vi "TA Main.vi"() -> ()   [LabVIEW 2019]
doc: "This example demonstrates how to acquire a continuous amount of data (Waveform) using the DAQ device's internal clock. It also shows how to synchronize two devices for different device families (E Series, S Series, M Series, X Series, DSA, and SC Express), to simultaneously acquire the data.\n\nFor instructions on how to connect your signals to the DAQ device, refer to your device documentation."
uses:
  <vilib>/Utility/error.llb/DialogType.ctl
  <vilib>/DAQmx/configure/trigger.llb/DAQmx Start Trigger (Digital Edge).vi
  <vilib>/DAQmx/read.llb/DAQmx Read (Analog 1D Wfm NChan NSamp).vi
  <vilib>/DAQmx/configure/timing.llb/DAQmx Timing (Sample Clock).vi
  <vilib>/Instr/_visa.llb/VISA Configure Serial Port (Instr).vi
  Program Files/National Instruments/LabVIEW 2019/examples/Instrument IO/Serial/support/Serial - Settings.ctl
panel:
  in  "Pass Logger":T1(tab)
  out "CO2 chart":waveform(dbl)[](graph)=[{"t0"=timestamp(3654846988.5963 s since 1904-01-01), "dt"=0.0, "Y"=[566.0], "attributes"=variant("NI_ChannelName"=variant(string "SCD30 CO2"), "NI_UnitDescription"=variant(string "ppm"))}, {"t0"=timestamp(3654846988.5963 s since 1904-01-01), "dt"=0.0, "Y"=[28.99], "attributes"=variant("NI_ChannelName"=variant(string "SCD30 Temp"), "NI_UnitDescription"=variant(string "C"))}, {"t0"=timestamp(3654846988.5963 s since 1904-01-01), "dt"=0.0, "Y"=[22.24], "attributes"=variant("NI_ChannelName"=variant(string "SCD30 Humidity"), "NI_UnitDescription"=variant(string "%"))}, {"t0"=timestamp(3654846988.5963 s since 1904-01-01), "dt"=0.0, "Y"=[28.2], "attributes"=variant("NI_ChannelName"=variant(string "BME680 Temp"), "NI_UnitDescription"=variant(string "C"))}, {"t0"=timestamp(3654846988.5963 s since 1904-01-01), "dt"=0.0, "Y"=[1011.41], "attributes"=variant("NI_ChannelName"=variant(string "hPa"), "NI_UnitDescription"=variant(string "BME680 Pressure"))}, {"t0"=timestamp(3654846988.5963 s since 1904-01-01), "dt"=0.0, "Y"=[23.86], "attributes"=variant("NI_ChannelName"=variant(string "BME680 Humidity"), "NI_UnitDescription"=variant(string "%"))}, {"t0"=timestamp(3654846988.5963 s since 1904-01-01), "dt"=0.0, "Y"=[407.63], "attributes"=variant("NI_ChannelName"=variant(string "BME680 Gas"), "NI_UnitDescription"=variant(string "KOhms"))}]
  in  "Stop":bool
  in  "Enable logging":bool=TRUE caption="Enable"
  in  "File config":T2={"Filepath"=path "C:/Users/Administrator/Desktop/DAQ PAS/Test data", "Test ID"="CO2_oven_V3_1v2_25C", "PC"="69DTQV2"}
  out "Lockin chart":waveform(dbl)[](graph)=[{"t0"=timestamp(3654846973.919467 s since 1904-01-01), "dt"=9.999, "Y"=[0.5432839233173321], "attributes"=variant("NI_ChannelName"=variant(string "Phase - Mic Diff"), "NI_UnitDescription"=variant(string "Rad"))}, {"t0"=timestamp(3654846973.919467 s since 1904-01-01), "dt"=9.999, "Y"=[0.28139672074027666], "attributes"=variant("NI_ChannelName"=variant(string "Amplitude - Mic Diff"), "NI_UnitDescription"=variant(string "Volts"))}]
  out "Lockin output 1":T3={"X"=0.12044000212072635, "Y"=0.07273399824019537, "R"=0.14069836037013833, "θ"=0.5432839233173321, "Amp"=0.28139672074027666, "dt"=9.999, "Active channel"="Mic Diff", "Ref channel"="Heater Voltage"} {"X" format="%#_3g"; "Y" format="%#_3g"; "R" format="%#_3g"}
  out "Reference sesnsor readings":T4={"SCD30 CO2"=566.0, "SCD30 Temp (C)"=28.99, "SCD30 RH (%)"=22.24, "BME680 Temp (C) "=28.2, "BME680 Presssure (hPa)"=1011.41, "BME680 RH (%) "=23.86, "BME680 Gas (KOhms)"=407.63}
  in  "Sampling config":cluster{"Fs":dbl, "#s":dbl}={"Fs"=1000.0, "#s"=10000.0} {"Fs" format="%.2p"}
  in  "Config 1":cluster{"Ref Index":i32, "Active Index":i32}={"Ref Index"=2, "Active Index"=4}
  out "Lockin output 5":T3={"X"=4.105476127421498, "Y"=0.07771898305094777, "R"=4.106211693660507, "θ"=0.018928304216159014, "Amp"=8.212423387321014, "dt"=9.999, "Active channel"="Heater Current", "Ref channel"="Heater Voltage"} {"X" format="%#_3g"; "Y" format="%#_3g"; "R" format="%#_3g"}
  out "Lockin output 6":T3={"X"=5.873296336618479, "Y"=0.05854532299570415, "R"=5.873588120781088, "θ"=0.009967721820028476, "Amp"=11.747176241562176, "dt"=9.999, "Active channel"="Heater Power", "Ref channel"="Heater Voltage"} {"X" format="%#_3g"; "Y" format="%#_3g"; "R" format="%#_3g"}
  out "Lockin output 4":T3={"X"=0.31867008645671724, "Y"=3.873316981852211e-05, "R"=0.31867008881065395, "θ"=0.00012154629905321044, "Amp"=0.6373401776213079, "dt"=9.999, "Active channel"="Heater Voltage", "Ref channel"="Heater Voltage"} {"X" format="%#_3g"; "Y" format="%#_3g"; "R" format="%#_3g"}
  out "Lockin output 3":T3={"X"=-0.12845683117209084, "Y"=-0.046514562917248106, "R"=0.1366190398083579, "θ"=-2.7941768834347642, "Amp"=0.2732380796167158, "dt"=9.999, "Active channel"="Mic Active", "Ref channel"="Heater Voltage"} {"X" format="%#_3g"; "Y" format="%#_3g"; "R" format="%#_3g"}
  out "Lockin output 2":T3={"X"=-0.008448931381000458, "Y"=0.02761458480398332, "R"=0.02887818788250469, "θ"=1.8677111087244906, "Amp"=0.05775637576500938, "dt"=9.999, "Active channel"="Mic Ref", "Ref channel"="Heater Voltage"} {"X" format="%#_3g"; "Y" format="%#_3g"; "R" format="%#_3g"}
  in  "Config 5":cluster{"Ref Index":i32, "Active Index":i32}={"Ref Index"=2, "Active Index"=5}
  in  "Config 4":cluster{"Ref Index":i32, "Active Index":i32}={"Ref Index"=2, "Active Index"=2}
  in  "Config 3":cluster{"Ref Index":i32, "Active Index":i32}={"Ref Index"=2, "Active Index"=1}
  in  "Config 2":cluster{"Ref Index":i32, "Active Index":i32}={"Ref Index"=2, "Active Index"=0}
  in  "Config 6":cluster{"Ref Index":i32, "Active Index":i32}={"Ref Index"=2, "Active Index"=7}
  out "Lockin output 1":T3={"X"=0.12044000212072635, "Y"=0.07273399824019537, "R"=0.14069836037013833, "θ"=0.5432839233173321, "Amp"=0.28139672074027666, "dt"=9.999, "Active channel"="Mic Diff", "Ref channel"="Heater Voltage"} {"X" format="%#_3g"; "Y" format="%#_3g"; "R" format="%#_3g"}
  in  "Config 7":cluster{"Ref Index":i32, "Active Index":i32}={"Ref Index"=2, "Active Index"=6}
  out "Lockin output 7":T3={"X"=7.678486794988711, "Y"=-0.3885980124293869, "R"=7.6883137212317285, "θ"=-0.05056553039103557, "Amp"=15.376627442463457, "dt"=9.999, "Active channel"="Heater Resistance", "Ref channel"="Heater Voltage"} {"X" format="%#_3g"; "Y" format="%#_3g"; "R" format="%#_3g"}
  in  "VISA resource name 2":refnum<visa-resource-name>="COM6"
  in  "Serial Settings":T5={"baud rate"=9600, "data bits"=8, "parity"=enum."None", "stop bits"=10, "flow control"=0} {"flow control" items=["None"=0, "XON/XOFF"=1, "RTS/CTS"=2, "DTR/DSR"=4]; "stop bits" items=["1.0"=10, "1.5"=15, "2.0"=20]; "data bits" min=5 max=8 step=1; "baud rate" items=["75"=75, "110"=110, "134"=134, "150"=150, "300"=300, "600"=600, "1200"=1200, "1800"=1800, "2400"=2400, "4800"=4800, "7200"=7200, "9600"=9600, "14400"=14400, "19200"=19200, "28800"=28800, "38400"=38400, "56000"=56000, "57600"=57600, "115200"=115200, "128000"=128000, "230400"=230400]}
  out "Waveform":waveform(dbl)(graph)={"t0"=timestamp(3654846973.919445 s since 1904-01-01), "dt"=0.001, "Y"=array[10000 elements], "attributes"=variant("NI_ChannelName"=variant(string "Mic Diff"), "NI_UnitDescription"=variant(string "Volts"))}
  out "Channel names":T6={"Ref channel"="Mic Ref", "Active channel"="Mic Active"}
  in  "Config":T7={"Ref Index"=0, "Active Index"=1, "Gain"=0.95, "Channel name"="Mic Diff", "Enable"=TRUE, "Offset"=0.0}
  in  "Channel config":T8={"Frequency"=70.0, "Voltage"=1.0, "Signal type"=enum."Sine Wave", "Square wave duty cycle (%)"=50.0, "physical channels"="Dev1/ao0", "name to assign"="Heater Voltage", "Offset (V)"=0.05} {"Square wave duty cycle (%)" format="%0.2f"}
  in  "Config":T9={"Voltage channel index"=2, "Shunt channel index"=3, "Shunt resistance"=10}
  out "Channel names":T10={"Voltage channel name"="Heater Voltage", "Shunt channel name"="Heater Shunt"}
  out "Microphone Waveform":waveform(dbl)[](graph)=[{"t0"=timestamp(3654846973.919445 s since 1904-01-01), "dt"=0.001, "Y"=array[10000 elements], "attributes"=variant("NI_ChannelName"=variant(string "Mic Ref"), "NI_UnitDescription"=variant(string "Volts"))}, {"t0"=timestamp(3654846973.919456 s since 1904-01-01), "dt"=0.001, "Y"=array[10000 elements], "attributes"=variant("NI_ChannelName"=variant(string "Mic Active"), "NI_UnitDescription"=variant(string "Volts"))}, {"t0"=timestamp(3654846973.919467 s since 1904-01-01), "dt"=0.001, "Y"=array[10000 elements], "attributes"=variant("NI_ChannelName"=variant(string "Heater Voltage"), "NI_UnitDescription"=variant(string "Volts"))}, {"t0"=timestamp(3654846973.919478 s since 1904-01-01), "dt"=0.001, "Y"=array[10000 elements], "attributes"=variant("NI_ChannelName"=variant(string "Heater Shunt"), "NI_UnitDescription"=variant(string "Volts"))}, {"t0"=timestamp(3654846973.919445 s since 1904-01-01), "dt"=0.001, "Y"=array[10000 elements], "attributes"=variant("NI_ChannelName"=variant(string "Mic Diff"), "NI_UnitDescription"=variant(string "Volts"))}, {"t0"=timestamp(3654846973.919478 s since 1904-01-01), "dt"=0.001, "Y"=array[10000 elements], "attributes"=variant("NI_ChannelName"=variant(string "Heater Current"), "NI_UnitDescription"=variant(string "mA"))}, {"t0"=timestamp(3654846973.919467 s since 1904-01-01), "dt"=0.001, "Y"=array[10000 elements], "attributes"=variant("NI_ChannelName"=variant(string "Heater Resistance"), "NI_UnitDescription"=variant(string "Ohms"))}, {"t0"=timestamp(3654846973.919467 s since 1904-01-01), "dt"=0.001, "Y"=array[10000 elements], "attributes"=variant("NI_ChannelName"=variant(string "Heater Power"), "NI_UnitDescription"=variant(string "mW"))}]
  out "Heater Waveform":waveform(dbl)[](graph)=[{"t0"=timestamp(3654846973.919445 s since 1904-01-01), "dt"=0.001, "Y"=array[10000 elements], "attributes"=variant("NI_ChannelName"=variant(string "Mic Ref"), "NI_UnitDescription"=variant(string "Volts"))}, {"t0"=timestamp(3654846973.919456 s since 1904-01-01), "dt"=0.001, "Y"=array[10000 elements], "attributes"=variant("NI_ChannelName"=variant(string "Mic Active"), "NI_UnitDescription"=variant(string "Volts"))}, {"t0"=timestamp(3654846973.919467 s since 1904-01-01), "dt"=0.001, "Y"=array[10000 elements], "attributes"=variant("NI_ChannelName"=variant(string "Heater Voltage"), "NI_UnitDescription"=variant(string "Volts"))}, {"t0"=timestamp(3654846973.919478 s since 1904-01-01), "dt"=0.001, "Y"=array[10000 elements], "attributes"=variant("NI_ChannelName"=variant(string "Heater Shunt"), "NI_UnitDescription"=variant(string "Volts"))}, {"t0"=timestamp(3654846973.919445 s since 1904-01-01), "dt"=0.001, "Y"=array[10000 elements], "attributes"=variant("NI_ChannelName"=variant(string "Mic Diff"), "NI_UnitDescription"=variant(string "Volts"))}, {"t0"=timestamp(3654846973.919478 s since 1904-01-01), "dt"=0.001, "Y"=array[10000 elements], "attributes"=variant("NI_ChannelName"=variant(string "Heater Current"), "NI_UnitDescription"=variant(string "mA"))}, {"t0"=timestamp(3654846973.919467 s since 1904-01-01), "dt"=0.001, "Y"=array[10000 elements], "attributes"=variant("NI_ChannelName"=variant(string "Heater Resistance"), "NI_UnitDescription"=variant(string "Ohms"))}, {"t0"=timestamp(3654846973.919467 s since 1904-01-01), "dt"=0.001, "Y"=array[10000 elements], "attributes"=variant("NI_ChannelName"=variant(string "Heater Power"), "NI_UnitDescription"=variant(string "mW"))}]
  in  "Channel 4 config":T11={"Channel"="Dev1/ai3", "Vmax"=0.5, "Vmin"=0.0, "name to assign"="Heater Shunt", "input terminal configuration"=10106} {"input terminal configuration" items=["Default"=-1, "RSE"=10083, "NRSE"=10078, "Differential"=10106, "Pseudodifferential"=12529]; "Vmin" format="%0.2f"; "Vmax" format="%0.2f"}
  in  "Channel 3 config":T11={"Channel"="Dev1/ai2", "Vmax"=3.0, "Vmin"=0.0, "name to assign"="Heater Voltage", "input terminal configuration"=10106} {"input terminal configuration" items=["Default"=-1, "RSE"=10083, "NRSE"=10078, "Differential"=10106, "Pseudodifferential"=12529]; "Vmin" format="%0.2f"; "Vmax" format="%0.2f"}
  in  "Channel 2 config":T11={"Channel"="Dev1/ai1", "Vmax"=3.0, "Vmin"=-3.0, "name to assign"="Mic Active", "input terminal configuration"=10083} {"input terminal configuration" items=["Default"=-1, "RSE"=10083, "NRSE"=10078, "Differential"=10106, "Pseudodifferential"=12529]; "Vmin" format="%0.2f"; "Vmax" format="%0.2f"}
  in  "Channel 1 config":T11={"Channel"="Dev1/ai0", "Vmax"=3.0, "Vmin"=-3.0, "name to assign"="Mic Ref", "input terminal configuration"=10083} {"input terminal configuration" items=["Default"=-1, "RSE"=10083, "NRSE"=10078, "Differential"=10106, "Pseudodifferential"=12529]; "Vmin" format="%0.2f"; "Vmax" format="%0.2f"}
  # "PAS Logger"
  # "(ppm)"
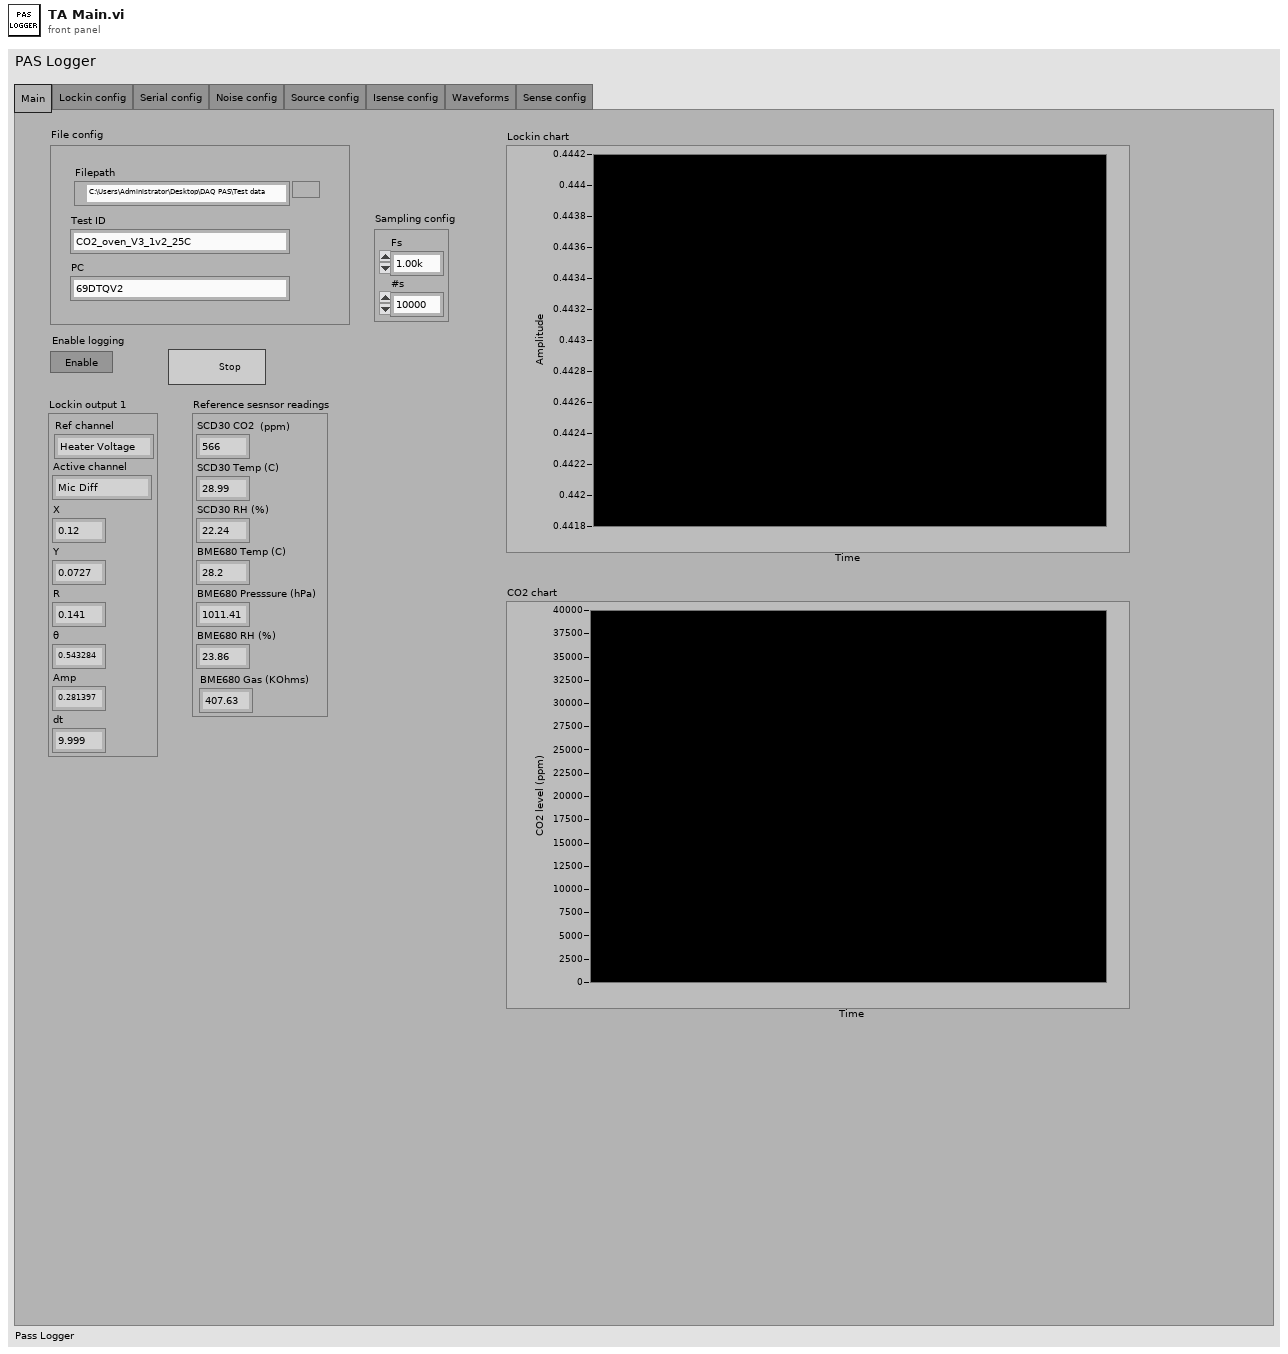
[diagram p1: front panel]
types:
  T1 = enum32{"Main", "Lockin config", "Serial config", "Noise config", "Source config", "Isense config", "Waveforms", "Sense config"}
  T2 = cluster{"Filepath":path, "Test ID":string, "PC":string}
  T3 = cluster{"X":dbl, "Y":dbl, "R":dbl, "θ":dbl, "Amp":dbl, "dt":dbl, "Active channel":string, "Ref channel":string}
  T4 = cluster{"SCD30 CO2":dbl, "SCD30 Temp (C)":dbl, "SCD30 RH (%)":dbl, "BME680 Temp (C) ":dbl, "BME680 Presssure (hPa)":dbl, "BME680 RH (%) ":dbl, "BME680 Gas (KOhms)":dbl}
  T5 = typedef "Serial - Settings.ctl" = cluster{"baud rate":u32, "data bits":u16, "parity":enum16{"None", "Odd", "Even", "Mark", "Space"}, "stop bits":u16, "flow control":u16}
  T6 = cluster{"Ref channel":string, "Active channel":string}
  T7 = cluster{"Ref Index":i32, "Active Index":i32, "Gain":dbl, "Channel name":string, "Enable":bool, "Offset":dbl}
  T8 = cluster{"Frequency":dbl, "Voltage":dbl, "Signal type":enum16{"Sine Wave", "Triangle Wave", "Square Wave", "Sawtooth Wave"}, "Square wave duty cycle (%)":dbl, "physical channels":tag, "name to assign":string, "Offset (V)":dbl}
  T9 = cluster{"Voltage channel index":i32, "Shunt channel index":i32, "Shunt resistance":i32}
  T10 = cluster{"Voltage channel name":string, "Shunt channel name":string}
  T11 = cluster{"Channel":tag, "Vmax":dbl, "Vmin":dbl, "name to assign":string, "input terminal configuration":i32}
  T12 = cluster{"Active channel":string, "Ref channel":string}
  T13 = typedef "DialogType.ctl" = u16
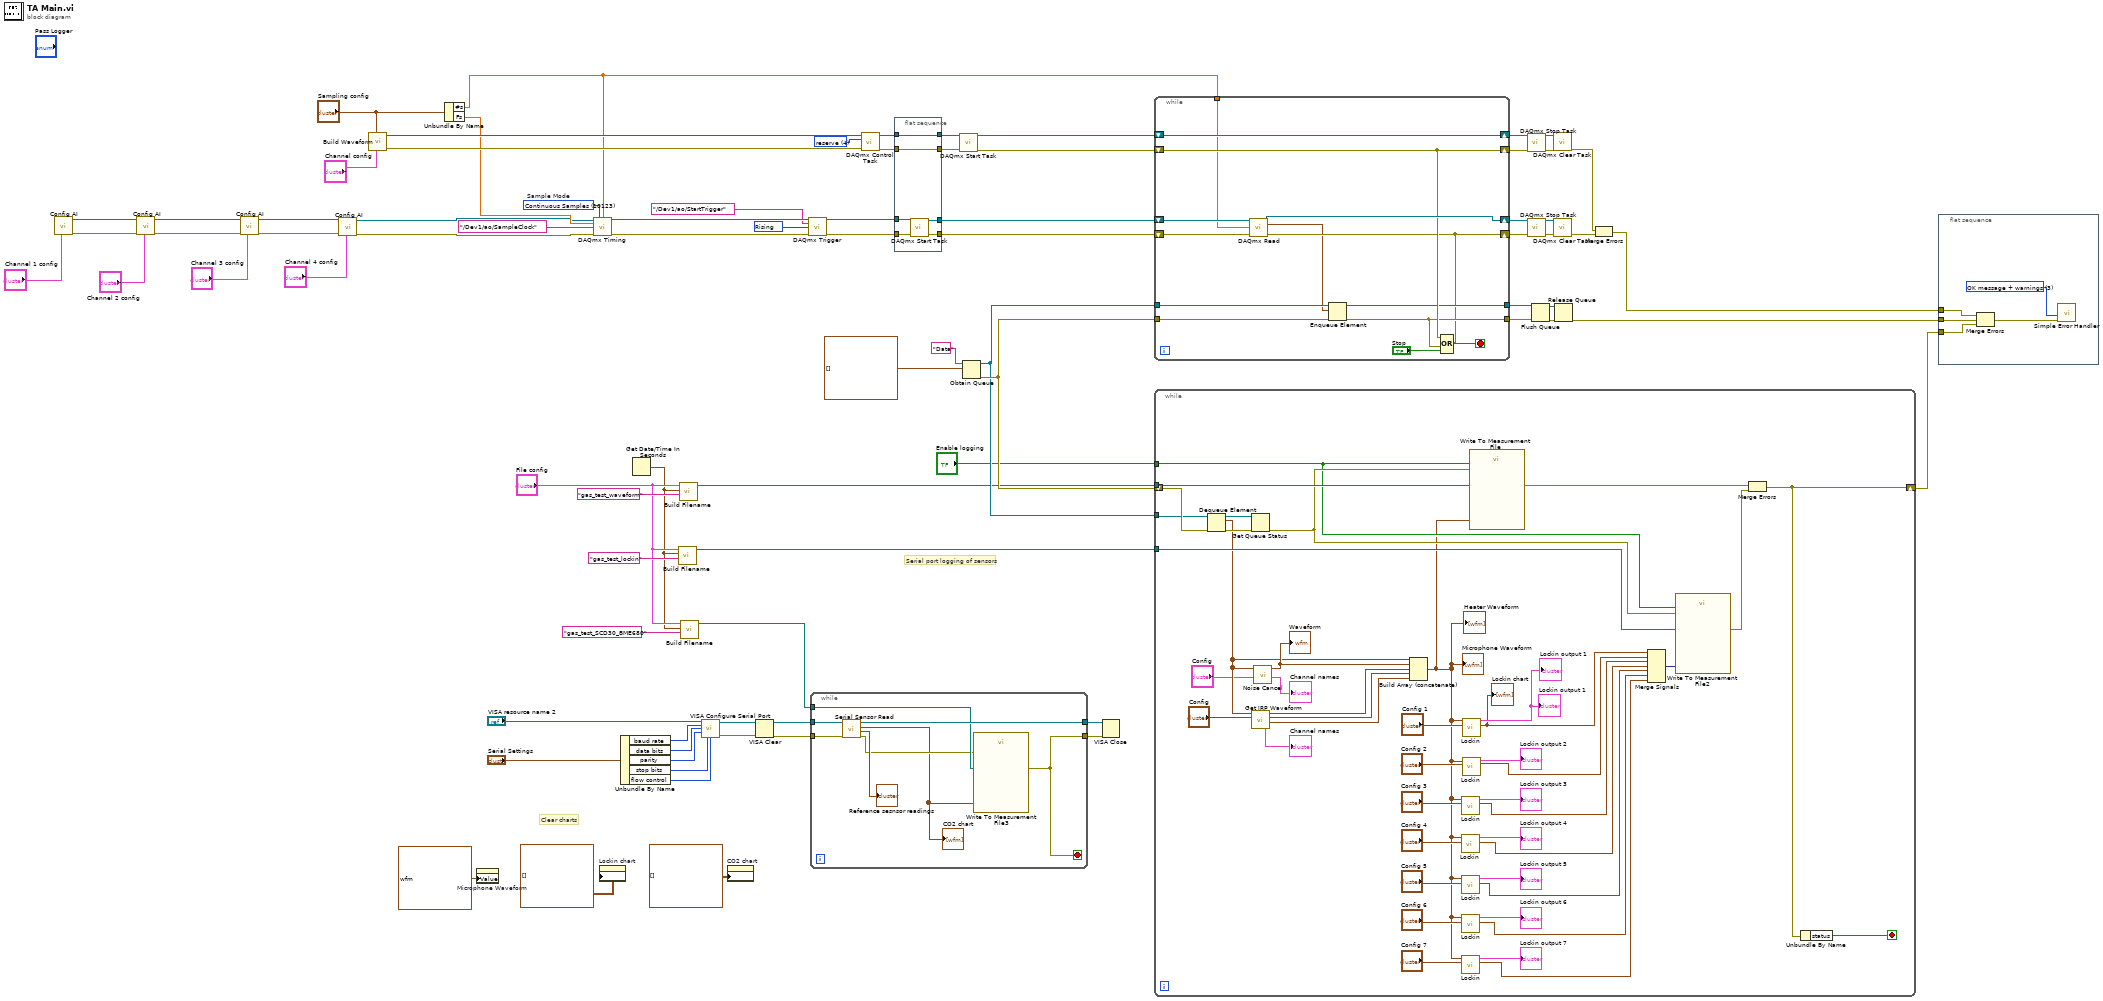
[diagram p0: block diagram]
diagram:
  w63 = 10280 items=["Rising"=10280, "Falling"=10171] ("edge")
  w70 = 4 items=["verify"=2, "reserve"=4, "commit"=3, "unreserve"=5, "abort"=6] ("action")
  w71 = 10123 items=["Finite Samples"=10178, "Continuous Samples"=10123, "Hardware Timed Single Point"=12522]  # Sample Mode
  # "Clear charts"
  # "Serial port logging of sensors"
  n1 = call "Config AI.vi"("Channel config"="Channel 1 config") -> ("error out"=w54:errorcluster, "task out"=w53:refnum<k21>)  [unwired: 9 in]
  n2 = call "Config AI.vi"("Channel config"="Channel 2 config", "error in"=w54, "task in"=w53) -> ("error out"=w3:errorcluster, "task out"=w2:refnum<k21>)  [unwired: 7 in]
  n3 = call "Config AI.vi"("Channel config"="Channel 3 config", "error in"=w3, "task in"=w2) -> ("error out"=w37:errorcluster, "task out"=w36:refnum<k21>)  [unwired: 7 in]
  n4 = call "Config AI.vi"("Channel config"="Channel 4 config", "error in"=w37, "task in"=w36) -> ("error out"=w35:errorcluster, "task out"=w34:refnum<k21>)  [unwired: 7 in]
  n5 = call "Build Waveform.vi"("sampling config"="Channel config", 7:"Sampling config") -> ("error out"=w52:errorcluster, "Waveform"=w51:waveform(dbl))  [unwired: 8 in]
  n6 = Unbundle By Name("Sampling config") -> ("#s"=w39:dbl, "Fs"=w38:dbl)
  n7 = property on="Microphone Waveform" class="WFGraph (strict)"("Value"=waveform(dbl)[] [{"t0"=timestamp(3651561790.263236 s since 1904-01-01), "dt"=0.001, "Y"=array[2000 elements], "attributes"=variant("NI_ChannelName"=variant(string "Mic Active"), "NI_UnitDescription"=variant(string "Volts"))}, {"t0"=timestamp(3651561790.263247 s since 1904-01-01), "dt"=0.001, "Y"=array[2000 elements], "attributes"=variant("NI_ChannelName"=variant(string "Mic Ref"), "NI_UnitDescription"=variant(string "Volts"))}, {"t0"=timestamp(3651561790.263258 s since 1904-01-01), "dt"=0.001, "Y"=array[2000 elements], "attributes"=variant("NI_ChannelName"=variant(string "Diode Heater"), "NI_UnitDescription"=variant(string "Volts"))}, {"t0"=timestamp(3651561790.263269 s since 1904-01-01), "dt"=0.001, "Y"=array[2000 elements], "attributes"=variant("NI_ChannelName"=variant(string "Diode Amb"), "NI_UnitDescription"=variant(string "Volts"))}, {"t0"=timestamp(3651561790.26328 s since 1904-01-01), "dt"=0.001, "Y"=array[2000 elements], "attributes"=variant("NI_ChannelName"=variant(string "Heater Shunt"), "NI_UnitDescription"=variant(string "Volts"))}, {"t0"=timestamp(3651561790.2632914 s since 1904-01-01), "dt"=0.001, "Y"=array[2000 elements], "attributes"=variant("NI_ChannelName"=variant(string "Heater V"), "NI_UnitDescription"=variant(string "Volts"))}, {"t0"=timestamp(3651561790.263247 s since 1904-01-01), "dt"=0.001, "Y"=array[2000 elements], "attributes"=variant("NI_ChannelName"=variant(string "Mic Diff"), "NI_UnitDescription"=variant(string "Volts"))}, {"t0"=timestamp(3651561790.26328 s since 1904-01-01), "dt"=0.001, "Y"=array[2000 elements], "attributes"=variant("NI_ChannelName"=variant(string "Heater Current"), "NI_UnitDescription"=variant(string "Amps"))}] ("Waveform")) -> ()  [unwired: 2 in, 2 out]
  n8 = call-poly <vilib>:"DAQmx Timing.vi"("task/channels in"=w34, "sample mode"=w71, "samples per channel"=w39, "rate"=w38, "source"=tag "/Dev1/ao/SampleClock", "error in"=w35) -> ("task out"=w64:refnum<k21>, "error out"=w65:errorcluster)  [unwired: 8 in]
  n9 = property on="Lockin chart" class="WFChart (strict)"("History Data"=waveform(dbl)[][] []) -> ()  [unwired: 2 in, 2 out]
  n10 = Unbundle By Name("Serial Settings") -> ("baud rate"=w18:u32, "data bits"=w17:u16, "parity"=w16:enum16{"None", "Odd", "Even", "Mark", "Space"}, "stop bits"=w15:u16, "flow control"=w14:u16)
  n11 = Get Date/Time In Seconds() -> (seconds since 1Jan1904=w21:timestamp)
  n12 = call "Build Filename.vi"("Test type"="gas_test_lockin" ("File Descriptor"), "time stamp"=w21, "File config"="File config") -> ("appended path"=w24:path)  [unwired: 8 in]
  n13 = call "Build Filename.vi"("Test type"="gas_test_waveform" ("File type"), "time stamp"=w21, "File config"="File config") -> ("appended path"=w26:path)  [unwired: 8 in]
  n14 = call "Build Filename.vi"("Test type"="gas_test_SCD30_BME680" ("File Descriptor"), "time stamp"=w21, "File config"="File config") -> ("appended path"=w7:path)  [unwired: 8 in]
  n15 = call-poly "VISA Configure Serial Port"("VISA resource name"="VISA resource name 2", "baud rate (9600)"=w18, "data bits (8)"=w17, "parity (0:none)"=w16, "stop bits (10: 1 bit)"=w15, "flow control (0:none)"=w14) -> ("VISA resource name out"=w12:refnum<visa-resource-name>, "error out"=w13:errorcluster)  [unwired: 3 in, 5 out]
  n16 = property on="CO2 chart" class="WFChart (strict)"("History Data"=waveform(dbl)[][] []) -> ()  [unwired: 2 in, 2 out]
  n17 = VISA Clear(VISA resource name=w12, error in (no error)=w13) -> (VISA resource name out=w11:refnum<visa-resource-name>, error out=w10:errorcluster)
  n18 = call-poly <vilib>:"DAQmx Trigger.vi"("task/channels in"=w64, "source"=tag "/Dev1/ao/StartTrigger", "edge"=w63, "error in"=w65) -> ("task out"=w61:refnum<k21>, "error out"=w62:errorcluster)  [unwired: 10 in]
  n19 = while {
    tunnel: w11 -> [w89]
    tunnel: w10 -> [w88]
    tunnel: [w83] -> w9
    tunnel: [w87] -> w8
    tunnel: w7 -> [w85]
    stop <- w83 stop-if-true
    n20 = call "Serial Sensor Read.vi"("error in (no error)"=w88, "VISA resource name"=w89) -> ("error out"=w84:errorcluster, "Readings"=→"Reference sesnsor readings":T4, "appended array"=w82:waveform(dbl)[], "VISA resource name out"=w87:refnum<visa-resource-name>)  [unwired: 6 in]
    "CO2 chart" <- w82
    n21 = call "Write To Measurement File3"("Signals"=w82, "error in (no error)"=w84, "Filename"=w85) -> ("error out"=w83:errorcluster)  [unwired: 14 in, 2 out]
  }
  n22 = call <vilib>:"DAQmx Control Task.vi"("task/channels in"=w51, "action"=w70, "error in"=w52) -> ("task out"=w60:refnum<k21>, "error out"=w58:errorcluster)  [unwired: 11 in]
  n23 = flat-sequence {
    tunnel: [w95] -> w67
    tunnel: [w94] -> w66
    tunnel: w62 -> [w93]
    tunnel: w61 -> [w92]
    tunnel: w60 -> [w91]
    tunnel: [w91] -> w59
    tunnel: w58 -> [w90]
    tunnel: [w90] -> w57
    frame #0 {
      n24 = call <vilib>:"DAQmx Start Task.vi"("task/channels in"=w92, "error in"=w93) -> ("task out"=w94:refnum<k21>, "error out"=w95:errorcluster)  [unwired: 12 in]
    }
  }
  n25 = call <vilib>:"DAQmx Start Task.vi"("task/channels in"=w59, "error in"=w57) -> ("task out"=w68:refnum<k21>, "error out"=w69:errorcluster)  [unwired: 12 in]
  n26 = Obtain Queue(name (unnamed)="Data" ("名前（名前なし）"), element data type=waveform(dbl)[] [] ("data")) -> (queue out=w42:refnum<queue>, error out=w43:errorcluster)  [unwired: 3 in, 1 out]
  n27 = VISA Close(VISA resource name=w8, error in (no error)=w9) -> ()  [unwired: 1 out]
  n28 = while {
    tunnel: w42 -> [w138]
    shift-right: [w129] -> w41
    shift-left: w43 -> [w139]
    tunnel: w26 -> [w137]
    tunnel: "Enable logging" -> [w133]
    tunnel: w24 -> [w132]
    stop <- w125 stop-if-true
    n29 = Dequeue Element(queue=w138, error in (no error)=w139) -> (queue out=w135:refnum<queue>, element=w106:waveform(dbl)[], error out=w136:errorcluster)  [unwired: 1 in, 1 out]
    n30 = Get Queue Status(queue=w135, error in (no error)=w136) -> (error out=w134:errorcluster)  [unwired: 1 in, 7 out]
    n31 = call "Get IRP Waveform.vi"("Channel config"="Config", "array"=w106) -> ("Power waveform out"=w101:waveform(dbl), "Resistance waveform out"=w102:waveform(dbl), "Current waveform out"=w104:waveform(dbl), "Channel names"=→"Channel names":T10)  [unwired: 6 in]
    n32 = call "Noise Cancel.vi"("Config"="Config", "array"=w106) -> ("Channel names"=→"Channel names":T12, "waveform out"=w127:waveform(dbl))  [unwired: 8 in]
    "Waveform" <- w127
    n33 = Build Array (concatenate)(w106, w127, w104, w102, w101) -> (w97:waveform(dbl)[])
    "Microphone Waveform" <- w97
    "Heater Waveform" <- w97
    n34 = call "Lockin.vi"("Config"="Config 4", "array"=w97) -> ("Output waveform"=w121:waveform(dbl)[], "Lockin output"=→"Lockin output 4":T3)  [unwired: 8 in]
    n35 = call "Lockin.vi"("Config"="Config 3", "array"=w97) -> ("Output waveform"=w122:waveform(dbl)[], "Lockin output"=→"Lockin output 3":T3)  [unwired: 8 in]
    n36 = call "Lockin.vi"("Config"="Config 5", "array"=w97) -> ("Output waveform"=w120:waveform(dbl)[], "Lockin output"=→"Lockin output 5":T3)  [unwired: 8 in]
    n37 = call "Lockin.vi"("Config"="Config 6", "array"=w97) -> ("Output waveform"=w119:waveform(dbl)[], "Lockin output"=→"Lockin output 6":T3)  [unwired: 8 in]
    n38 = call "Lockin.vi"("Config"="Config 7", "array"=w97) -> ("Output waveform"=w96:waveform(dbl)[], "Lockin output"=→"Lockin output 7":T3)  [unwired: 8 in]
    n39 = call "Lockin.vi"("Config"="Config 1", "array"=w97) -> ("Output waveform"=w107:waveform(dbl)[], "Lockin output"=→"Lockin output 1" →"Lockin output 1":T3)  [unwired: 8 in]
    "Lockin chart" <- w107
    n40 = call "Lockin.vi"("Config"="Config 2", "array"=w97) -> ("Output waveform"=w123:waveform(dbl)[], "Lockin output"=→"Lockin output 2":T3)  [unwired: 8 in]
    n41 = call "Write To Measurement File"("Signals"=w97, "Enable"=w133, "error in (no error)"=w134, "Filename"=w137) -> ("error out"=w130:errorcluster)  [unwired: 13 in, 2 out]
    n42 = Merge Signals(w107, w123, w122, w121, w120, w119, w96) -> (w118:dynamicdata)
    n43 = call "Write To Measurement File2"("Signals"=w118, "Enable"=w133, "error in (no error)"=w134, "Filename"=w132) -> ("error out"=w131:errorcluster)  [unwired: 13 in, 2 out]
    n44 = Merge Errors(w130, w131) -> (w129:errorcluster)
    n45 = Unbundle By Name(w129) -> ("status"=w125:bool)
  }
  n46 = while {
    shift-right: [w149] -> w80
    shift-left: w69 -> [w149]
    shift-right: [w141] -> w76
    shift-left: w67 -> [w151]
    shift-right: [w148] -> w81
    shift-left: w68 -> [w148]
    shift-right: [w150] -> w77
    shift-left: w66 -> [w152]
    tunnel: w39 -> [w147]
    tunnel: [w146] -> w48
    tunnel: [w142] -> w47
    tunnel: w42 -> [w145]
    tunnel: w43 -> [w144]
    stop <- w153 stop-if-true
    n47 = call-poly <vilib>:"DAQmx Read.vi"("task/channels in"=w152, "number of samples per channel"=w147, "error in"=w151) -> ("task out"=w150:refnum<k21>, "data"=w140:waveform(dbl)[], "error out"=w141:errorcluster)  [unwired: 10 in]
    n48 = Enqueue Element(queue=w145, element=w140, error in (no error)=w144) -> (queue out=w146:refnum<queue>, error out=w142:errorcluster)  [unwired: 1 in, 1 out]
    n49 = Compound Arithmetic op=OR(w149, w141, w142, "Stop") -> (w153:bool)
  }
  n50 = call <vilib>:"DAQmx Stop Task.vi"("task/channels in"=w81, "error in"=w80) -> ("task out"=w78:refnum<k21>, "error out"=w79:errorcluster)  [unwired: 12 in]
  n51 = call <vilib>:"DAQmx Stop Task.vi"("task/channels in"=w77, "error in"=w76) -> ("task out"=w74:refnum<k21>, "error out"=w75:errorcluster)  [unwired: 12 in]
  n52 = Flush Queue(queue=w48, error in (no error)=w47) -> (queue out=w49:refnum<queue>, error out=w50:errorcluster)  [unwired: 1 out]
  n53 = call <vilib>:"DAQmx Clear Task.vi"("task in"=w78, "error in"=w79) -> ("error out"=w73:errorcluster)  [unwired: 13 in]
  n54 = call <vilib>:"DAQmx Clear Task.vi"("task in"=w74, "error in"=w75) -> ("error out"=w72:errorcluster)  [unwired: 13 in]
  n55 = Release Queue(queue=w49, error in (no error)=w50) -> (error out=w45:errorcluster)  [unwired: 1 in, 2 out]
  n56 = Merge Errors(w73, w72) -> (w46:errorcluster)
  n57 = flat-sequence {
    tunnel: w46 -> [w158]
    tunnel: w45 -> [w157]
    tunnel: w41 -> [w154]
    frame #0 {
      w156 = T13 3 items=["no dialog", "OK message", "continue or stop message", "OK message + warnings", "continue/stop + warnings"] ("type of dialog (OK msg:1)")
      n58 = Merge Errors(w158, w157, w154) -> (w155:errorcluster)
      n59 = call <vilib>:"Simple Error Handler.vi"("type of dialog (OK msg:1)"=w156, "error in (no error)"=w155) -> ()  [unwired: 3 in, 5 out]
    }
  }
